vi "find_new_centroid.vi"(9 "centroide (ponto, índice)":T1, 11 "Array":T2(array[cluster])) -> (3 "centroide (ponto, índice) 2":T1)   [LabVIEW 2016]
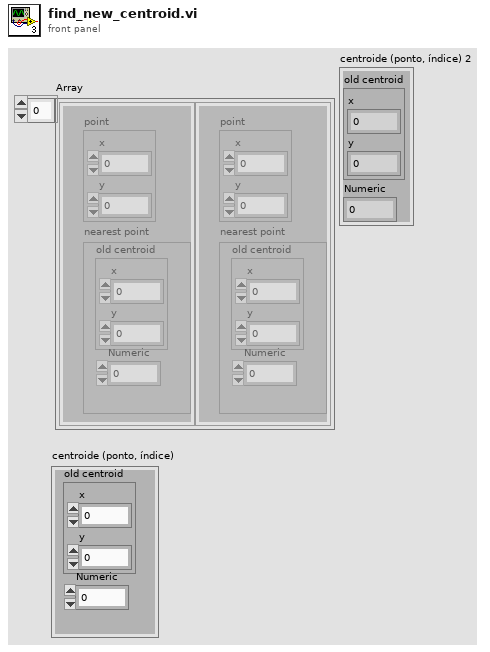
[diagram p1: front panel]
types:
  T1 = cluster{"old centroid":cluster{"x":dbl, "y":dbl}, "Numeric":i32}
  T2 = cluster{"point":cluster{"x":dbl, "y":dbl}, "nearest point":cluster{"old centroid":cluster{"x":dbl, "y":dbl}, "Numeric":i32}}[]
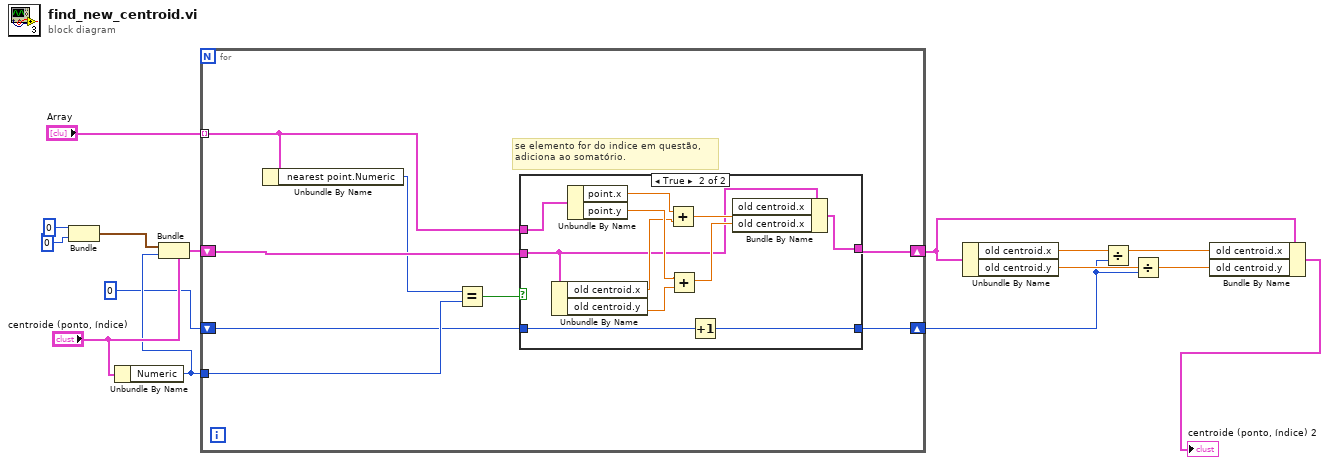
[diagram p0: block diagram]
diagram:
  n1 = Bundle(0, 0) -> (w11:cluster{i32, i32})  [unwired: 1 in]
  n2 = Unbundle By Name("centroide (ponto, índice)") -> ("Numeric"=w12:i32)
  n3 = Bundle(cluster="centroide (ponto, índice)", "old centroid"=w11, "Numeric"=w12) -> (w14:T1)
  n4 = for {
    shift-right: [w20] -> w7
    shift-left: w14 -> [w23]
    tunnel: "Array" -> [w22] mode=indexing
    tunnel: w12 -> [w21]
    shift-right: [w19] -> w1
    shift-left: 0 -> [w18]
    # "se elemento for do indice em questão,\nadiciona ao somatório."
    n5 = Unbundle By Name(w22) -> ("nearest point.Numeric"=w16:i32)
    n6 = Equal?(x=w16, y=w21) -> (x = y?=w17:bool)
    n7 = case shown="True" w17 {
      tunnel: [w25 w30] -> w20
      tunnel: w23 -> [w25 w28]
      tunnel: w22 -> [_ w29]
      tunnel: [w24 w26] -> w19
      tunnel: w18 -> [w24 w27]
      frame False {
      }
      frame True {
        n8 = Unbundle By Name(w28) -> ("old centroid.x"=w34:dbl, "old centroid.y"=w33:dbl)
        n9 = Unbundle By Name(w29) -> ("point.x"=w36:dbl, "point.y"=w35:dbl)
        n10 = Add(x=w36, y=w34) -> (x+y=w32:dbl)
        n11 = Add(x=w35, y=w33) -> (x+y=w31:dbl)
        n12 = Increment(x=w27) -> (x+1=w26:i32)
        n13 = Bundle By Name(cluster=w28, "old centroid.x"=w32, "old centroid.x"=w31) -> (w30:T1)
      }
    }
  }
  n14 = Unbundle By Name(w7) -> ("old centroid.x"=w6:dbl, "old centroid.y"=w2:dbl)
  n15 = Divide(x=w6, y=w1) -> (x/y=w4:dbl)
  n16 = Divide(x=w2, y=w1) -> (x/y=w3:dbl)
  n17 = Bundle By Name(cluster=w7, "old centroid.x"=w4, "old centroid.y"=w3) -> (→"centroide (ponto, índice) 2":T1)
